vi "Measure Settings Dialog.vi"(8 "error in (no error)":errorcluster caption="错误输入（无错误）", 10 "测试类型":T1, 11 "Settings in":T5={"Hardware Configuration"={"电压读取设置"={"DAQmx Channel"="", "Max Input"=0.0, "Min Input"=0.0, "Sample Rate"=0.0, "Sample Number"=0, "DAQmx Task"="", "device in"=""}, "角度传感器设置"={"counter"="Dev1/ctr0", "units"=10146, "分辨率"=0, "初始角度"=0.0, "DecodingType"=10092, "A相端口"="/Dev1/PFI8", "B相端口"="/Dev1/PFI8", "task in"=""}}, "Logging Configuration"={"Log File Base Path"=path "", "电压传感器转换率"=[], "电压传感器本底"=[]}, "Action Configuration"={"PLC设置"={"ActLogicalStationNumber"=9600, "ActUtlType"=refnum}, "动作设置"={"自动跳法测试动作"={"夹紧"={"PLC指令"={"变量类型"=2, "PLC地址"=0, "size"=0, "写入数据(写入时有效)"=0}}, "通油"={"打开主阀"={"变量类型"=2, "PLC地址"=0, "size"=0, "写入数据(写入时有效)"=0}, "打开电磁阀"={"变量类型"=2, "PLC地址"=0, "size"=0, "写入数据(写入时有效)"=0}}, "压销"={"PLC指令"={"变量类型"=2, "PLC地址"=0, "size"=0, "写入数据(写入时有效)"=0}}}, "其他动作"={"其他指令1"={"变量类型"=2, "PLC地址"=0, "size"=0, "写入数据(写入时有效)"=0}, "其他指令2"={"变量类型"=2, "PLC地址"=0, "size"=0, "写入数据(写入时有效)"=0}, "其他指令3"={"变量类型"=2, "PLC地址"=0, "size"=0, "写入数据(写入时有效)"=0}, "其他指令4"={"变量类型"=2, "PLC地址"=0, "size"=0, "写入数据(写入时有效)"=0}, "其他指令5"={"变量类型"=2, "PLC地址"=0, "size"=0, "写入数据(写入时有效)"=0}}}, "电机设置"={"counter"="Dev1/ctr0", "方向端口"="", "当前方向"=FALSE, "频率"=0.0, "DAQmx Task"=""}, "所有测试电机转动逻辑"={"啮合测试电机转动逻辑"={"反转判断条件1"={"传感器序号"=0, "条件"=enum."小于", "值"=0.0, "条件判断时间间隔"=0, "反转等待时长"=0}, "停止判断条件1"={"角度传感器序号"=0, "正转/反转"=enum."正转", "反转次数"=0, "停止角度"=0.0, "停止角度误差范围"=0.0}}, "退回测试电机转动逻辑"={"反转判断条件1"={"传感器序号"=0, "条件"=enum."小于", "值"=0.0, "条件判断时间间隔"=0, "反转等待时长"=0}, "停止判断条件1"={"角度传感器序号"=0, "正转/反转"=enum."正转", "反转次数"=0, "停止角度"=0.0, "停止角度误差范围"=0.0}}, "功能测试电机转动逻辑"={"反转判断条件1"={"传感器序号"=0, "条件"=enum."小于", "值"=0.0, "条件判断时间间隔"=0, "反转等待时长"=0}, "停止判断条件1"={"角度传感器序号"=0, "正转/反转"=enum."正转", "反转次数"=0, "停止角度"=0.0, "停止角度误差范围"=0.0}}, "力特性测试电机转动逻辑"={"反转判断条件1"={"传感器序号"=0, "条件"=enum."小于", "值"=0.0, "条件判断时间间隔"=0, "反转等待时长"=0}, "停止判断条件1"={"角度传感器序号"=0, "正转/反转"=enum."正转", "反转次数"=0, "停止角度"=0.0, "停止角度误差范围"=0.0}}, "自动调阀测试分中电机转动逻辑"={"反转判断条件1"={"传感器序号"=0, "条件"=enum."小于", "值"=0.0, "条件判断时间间隔"=0, "反转等待时长"=0}, "停止判断条件1"={"角度传感器序号"=0, "正转/反转"=enum."正转", "反转次数"=0, "停止角度"=0.0, "停止角度误差范围"=0.0}}, "自动调阀测试对中电机转动逻辑"={"反转判断条件1"={"传感器序号"=0, "条件"=enum."小于", "值"=0.0, "条件判断时间间隔"=0, "反转等待时长"=0}, "停止判断条件1"={"角度传感器序号"=0, "正转/反转"=enum."正转", "反转次数"=0, "停止角度"=0.0, "停止角度误差范围"=0.0}}}}} caption="设置" {"Action Configuration"."动作设置"."其他动作"."其他指令5"."变量类型" items=["X", "Y", "M", "D"]; "Action Configuration"."动作设置"."其他动作"."其他指令4"."变量类型" items=["X", "Y", "M", "D"]; "Action Configuration"."动作设置"."其他动作"."其他指令3"."变量类型" items=["X", "Y", "M", "D"]; "Action Configuration"."动作设置"."其他动作"."其他指令2"."变量类型" items=["X", "Y", "M", "D"]; "Action Configuration"."动作设置"."其他动作"."其他指令1"."变量类型" items=["X", "Y", "M", "D"]; "Action Configuration"."动作设置"."自动跳法测试动作"."压销"."PLC指令"."变量类型" items=["X", "Y", "M", "D"]; "Action Configuration"."动作设置"."自动跳法测试动作"."通油"."打开电磁阀"."变量类型" items=["X", "Y", "M", "D"]; "Action Configuration"."动作设置"."自动跳法测试动作"."通油"."打开主阀"."变量类型" items=["X", "Y", "M", "D"]; "Action Configuration"."动作设置"."自动跳法测试动作"."夹紧"."PLC指令"."变量类型" items=["X", "Y", "M", "D"]; "Hardware Configuration"."角度传感器设置"."DecodingType" items=["X1"=10090, "X2"=10091, "X4"=10092, "Two Pulse Counting"=10313]; "Hardware Configuration"."角度传感器设置"."units" items=["Degrees"=10146, "Radians"=10273, "Ticks"=10304, "From Custom Scale"=10065]}) -> (0 "error out":errorcluster caption="错误输出", 1 "Cancelled?":bool=TRUE caption="取消？", 2 "UI Refresh Needed?":bool caption="需要刷新UI？", 3 "Settings out":T5={"Hardware Configuration"={"电压读取设置"={"DAQmx Channel"="", "Max Input"=0.0, "Min Input"=0.0, "Sample Rate"=0.0, "Sample Number"=0, "DAQmx Task"="", "device in"=""}, "角度传感器设置"={"counter"="Dev1/ctr0", "units"=10146, "分辨率"=0, "初始角度"=0.0, "DecodingType"=10092, "A相端口"="/Dev1/PFI8", "B相端口"="/Dev1/PFI8", "task in"=""}}, "Logging Configuration"={"Log File Base Path"=path "", "电压传感器转换率"=[], "电压传感器本底"=[]}, "Action Configuration"={"PLC设置"={"ActLogicalStationNumber"=9600, "ActUtlType"=refnum}, "动作设置"={"自动跳法测试动作"={"夹紧"={"PLC指令"={"变量类型"=2, "PLC地址"=0, "size"=0, "写入数据(写入时有效)"=0}}, "通油"={"打开主阀"={"变量类型"=2, "PLC地址"=0, "size"=0, "写入数据(写入时有效)"=0}, "打开电磁阀"={"变量类型"=2, "PLC地址"=0, "size"=0, "写入数据(写入时有效)"=0}}, "压销"={"PLC指令"={"变量类型"=2, "PLC地址"=0, "size"=0, "写入数据(写入时有效)"=0}}}, "其他动作"={"其他指令1"={"变量类型"=2, "PLC地址"=0, "size"=0, "写入数据(写入时有效)"=0}, "其他指令2"={"变量类型"=2, "PLC地址"=0, "size"=0, "写入数据(写入时有效)"=0}, "其他指令3"={"变量类型"=2, "PLC地址"=0, "size"=0, "写入数据(写入时有效)"=0}, "其他指令4"={"变量类型"=2, "PLC地址"=0, "size"=0, "写入数据(写入时有效)"=0}, "其他指令5"={"变量类型"=2, "PLC地址"=0, "size"=0, "写入数据(写入时有效)"=0}}}, "电机设置"={"counter"="Dev1/ctr0", "方向端口"="", "当前方向"=FALSE, "频率"=0.0, "DAQmx Task"=""}, "所有测试电机转动逻辑"={"啮合测试电机转动逻辑"={"反转判断条件1"={"传感器序号"=0, "条件"=enum."小于", "值"=0.0, "条件判断时间间隔"=0, "反转等待时长"=0}, "停止判断条件1"={"角度传感器序号"=0, "正转/反转"=enum."正转", "反转次数"=0, "停止角度"=0.0, "停止角度误差范围"=0.0}}, "退回测试电机转动逻辑"={"反转判断条件1"={"传感器序号"=0, "条件"=enum."小于", "值"=0.0, "条件判断时间间隔"=0, "反转等待时长"=0}, "停止判断条件1"={"角度传感器序号"=0, "正转/反转"=enum."正转", "反转次数"=0, "停止角度"=0.0, "停止角度误差范围"=0.0}}, "功能测试电机转动逻辑"={"反转判断条件1"={"传感器序号"=0, "条件"=enum."小于", "值"=0.0, "条件判断时间间隔"=0, "反转等待时长"=0}, "停止判断条件1"={"角度传感器序号"=0, "正转/反转"=enum."正转", "反转次数"=0, "停止角度"=0.0, "停止角度误差范围"=0.0}}, "力特性测试电机转动逻辑"={"反转判断条件1"={"传感器序号"=0, "条件"=enum."小于", "值"=0.0, "条件判断时间间隔"=0, "反转等待时长"=0}, "停止判断条件1"={"角度传感器序号"=0, "正转/反转"=enum."正转", "反转次数"=0, "停止角度"=0.0, "停止角度误差范围"=0.0}}, "自动调阀测试分中电机转动逻辑"={"反转判断条件1"={"传感器序号"=0, "条件"=enum."小于", "值"=0.0, "条件判断时间间隔"=0, "反转等待时长"=0}, "停止判断条件1"={"角度传感器序号"=0, "正转/反转"=enum."正转", "反转次数"=0, "停止角度"=0.0, "停止角度误差范围"=0.0}}, "自动调阀测试对中电机转动逻辑"={"反转判断条件1"={"传感器序号"=0, "条件"=enum."小于", "值"=0.0, "条件判断时间间隔"=0, "反转等待时长"=0}, "停止判断条件1"={"角度传感器序号"=0, "正转/反转"=enum."正转", "反转次数"=0, "停止角度"=0.0, "停止角度误差范围"=0.0}}}}} caption="设置" {"Action Configuration"."动作设置"."其他动作"."其他指令5"."变量类型" items=["X", "Y", "M", "D"]; "Action Configuration"."动作设置"."其他动作"."其他指令4"."变量类型" items=["X", "Y", "M", "D"]; "Action Configuration"."动作设置"."其他动作"."其他指令3"."变量类型" items=["X", "Y", "M", "D"]; "Action Configuration"."动作设置"."其他动作"."其他指令2"."变量类型" items=["X", "Y", "M", "D"]; "Action Configuration"."动作设置"."其他动作"."其他指令1"."变量类型" items=["X", "Y", "M", "D"]; "Action Configuration"."动作设置"."自动跳法测试动作"."压销"."PLC指令"."变量类型" items=["X", "Y", "M", "D"]; "Action Configuration"."动作设置"."自动跳法测试动作"."通油"."打开电磁阀"."变量类型" items=["X", "Y", "M", "D"]; "Action Configuration"."动作设置"."自动跳法测试动作"."通油"."打开主阀"."变量类型" items=["X", "Y", "M", "D"]; "Action Configuration"."动作设置"."自动跳法测试动作"."夹紧"."PLC指令"."变量类型" items=["X", "Y", "M", "D"]; "Hardware Configuration"."角度传感器设置"."DecodingType" items=["X1"=10090, "X2"=10091, "X4"=10092, "Two Pulse Counting"=10313]; "Hardware Configuration"."角度传感器设置"."units" items=["Degrees"=10146, "Radians"=10273, "Ticks"=10304, "From Custom Scale"=10065]})   [LabVIEW 2015, in "Settings.lvlib"]
doc: "用于选择用户设置的对话框。"
uses:
  Settings.lvlib
  <vilib>/Utility/xml.llb/Write to XML File(string).vi
  Acquisition/Hardware Configuration.ctl
  Acquisition/Acquisition.lvlib
  Logging/Logging Configuration.ctl
  Logging/Logging.lvlib
  Settings.ctl
  Action/Action.lvlib
  Measure/Measure Type.ctl
  Action/Hardware Configuration.ctl
panel:
  in  "电机转动逻辑1":T2
  in  "Cancel Button":bool caption="取消按钮"
  in  "OK Button":bool caption="确定按钮"
  # "电机转动设置"
  # "对话框不可见部分（用于连线板）"
  # "1、扭矩\n\n2、油压\n\n3、左推力\n\n4、右推力\n\n5、流量\n\n6、位移量"
  # "1、扭矩\n\n2、油压\n\n3、左推力\n\n4、右推力\n\n5、流量\n\n6、位移量"
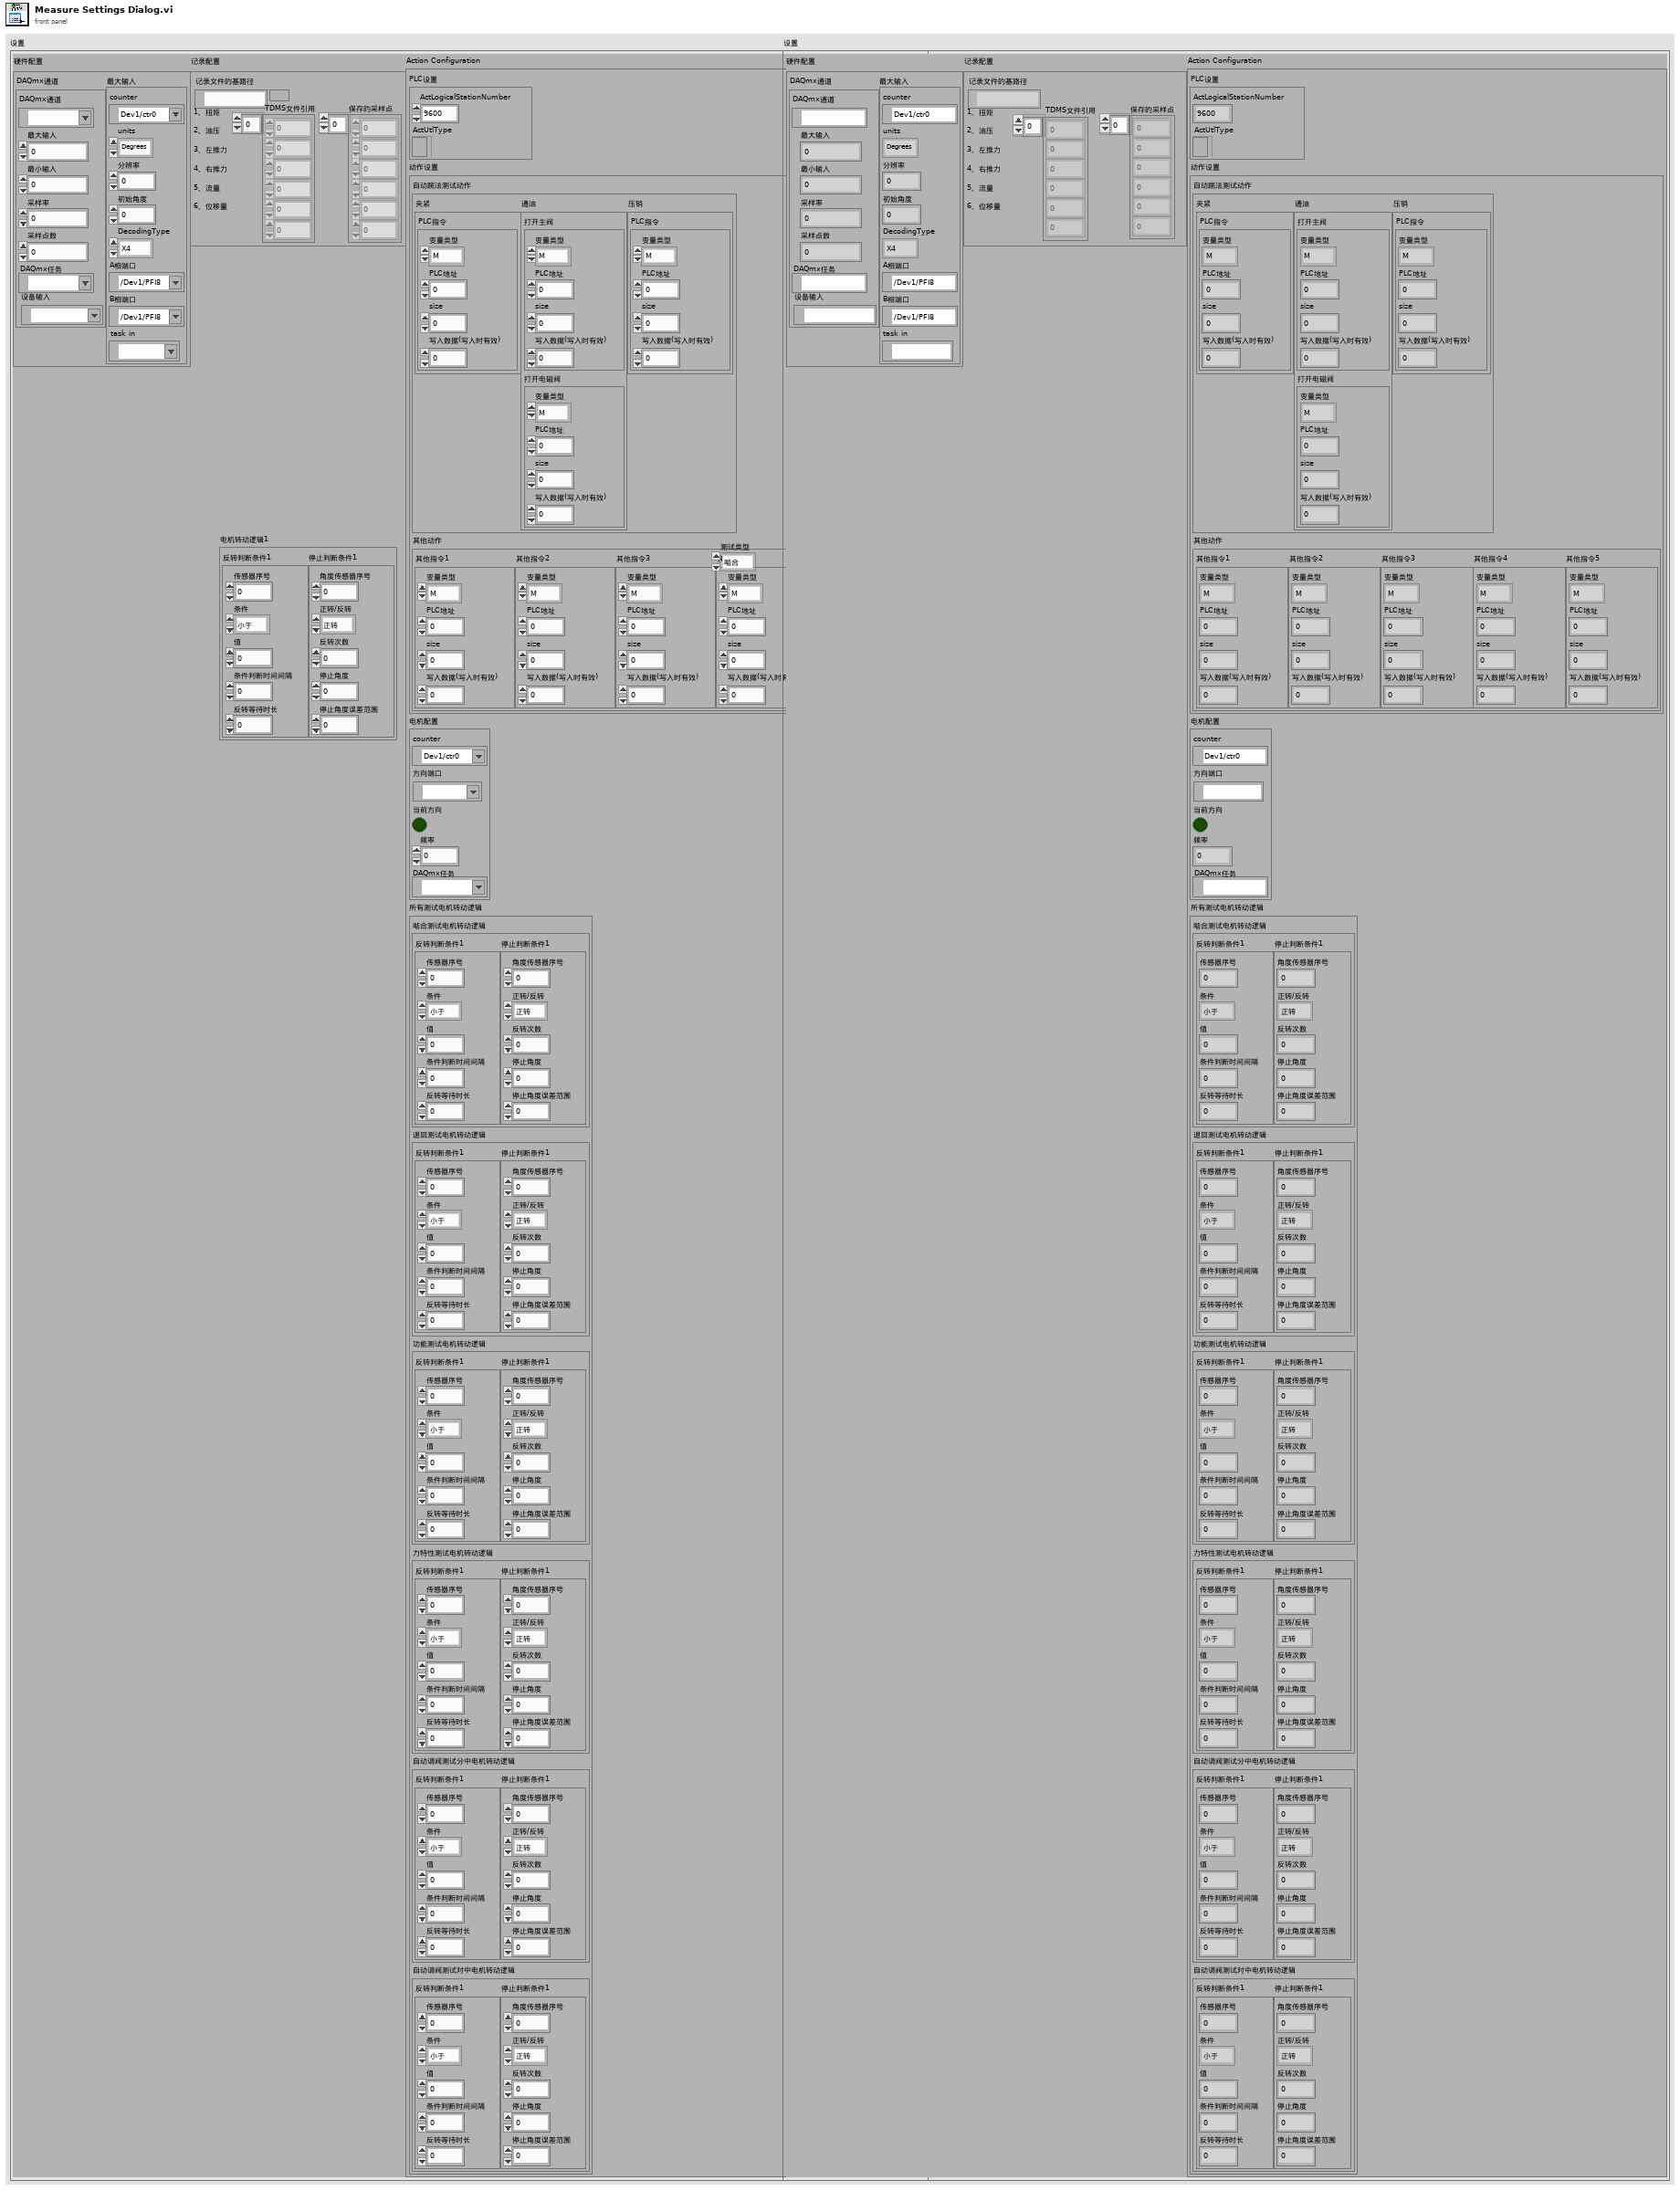
[diagram p1: front panel]
types:
  T1 = typedef "Measure Type.ctl" = enum16{"啮合", "退回", "功能", "力特性", "内泄漏", "自动调阀测试"}
  T2 = typedef "Action.lvlib/电机转动逻辑1.ctl" = cluster{"反转判断条件1":T3, "停止判断条件1":T4}
  T3 = typedef "Action.lvlib/反转判断条件1.ctl" = cluster{"传感器序号":i32, "条件":enum16{"小于", "大于", "等于"}, "值":dbl, "条件判断时间间隔":i32, "反转等待时长":i32}
  T4 = typedef "Action.lvlib/停止判断条件1.ctl" = cluster{"角度传感器序号":i32, "正转/反转":enum16{"正转", "反转"}, "反转次数":i32, "停止角度":dbl, "停止角度误差范围":dbl}
  T5 = typedef "Settings.lvlib/Settings.ctl" = cluster{"Hardware Configuration":T6, "Logging Configuration":T7, "Action Configuration":T8}
  T6 = typedef "Acquisition.lvlib/Hardware Configuration.ctl" = cluster{"电压读取设置":cluster{"DAQmx Channel":tag, "Max Input":dbl, "Min Input":dbl, "Sample Rate":dbl, "Sample Number":i32, "DAQmx Task":refnum<k21>, "device in":tag}, "角度传感器设置":cluster{"counter":tag, "units":i32, "分辨率":i32, "初始角度":dbl, "DecodingType":i32, "A相端口":tag, "B相端口":tag, "task in":refnum<k21>}}
  T7 = typedef "Logging.lvlib/Logging Configuration.ctl" = cluster{"Log File Base Path":path, "电压传感器转换率":dbl[], "电压传感器本底":dbl[]}
  T8 = typedef "Action.lvlib/Hardware Configuration.ctl" = cluster{"PLC设置":T9, "动作设置":T10, "电机设置":T14, "所有测试电机转动逻辑":T15}
  T9 = typedef "Action.lvlib/PLC设置.ctl" = cluster{"ActLogicalStationNumber":i32, "ActUtlType":refnum<k7>}
  T10 = typedef "Action.lvlib/动作设置.ctl" = cluster{"自动跳法测试动作":T11, "其他动作":T13}
  T11 = typedef "Action.lvlib/自动调阀测试动作设置.ctl" = cluster{"夹紧":cluster{"PLC指令":T12}, "通油":cluster{"打开主阀":T12, "打开电磁阀":T12}, "压销":cluster{"PLC指令":T12}}
  T12 = typedef "Action.lvlib/PLC控制指令.ctl" = cluster{"变量类型":u32, "PLC地址":i32, "size":i32, "写入数据(写入时有效)":i16}
  T13 = typedef "Action.lvlib/其他动作设置 .ctl" = cluster{"其他指令1":T12, "其他指令2":T12, "其他指令3":T12, "其他指令4":T12, "其他指令5":T12}
  T14 = typedef "Action.lvlib/电机控制设置.ctl" = cluster{"counter":tag, "方向端口":tag, "当前方向":bool, "频率":dbl, "DAQmx Task":refnum<k21>}
  T15 = typedef "Action.lvlib/所有测试电机转动逻辑.ctl" = cluster{"啮合测试电机转动逻辑":T2, "退回测试电机转动逻辑":T2, "功能测试电机转动逻辑":T2, "力特性测试电机转动逻辑":T2, "自动调阀测试分中电机转动逻辑":T2, "自动调阀测试对中电机转动逻辑":T2}
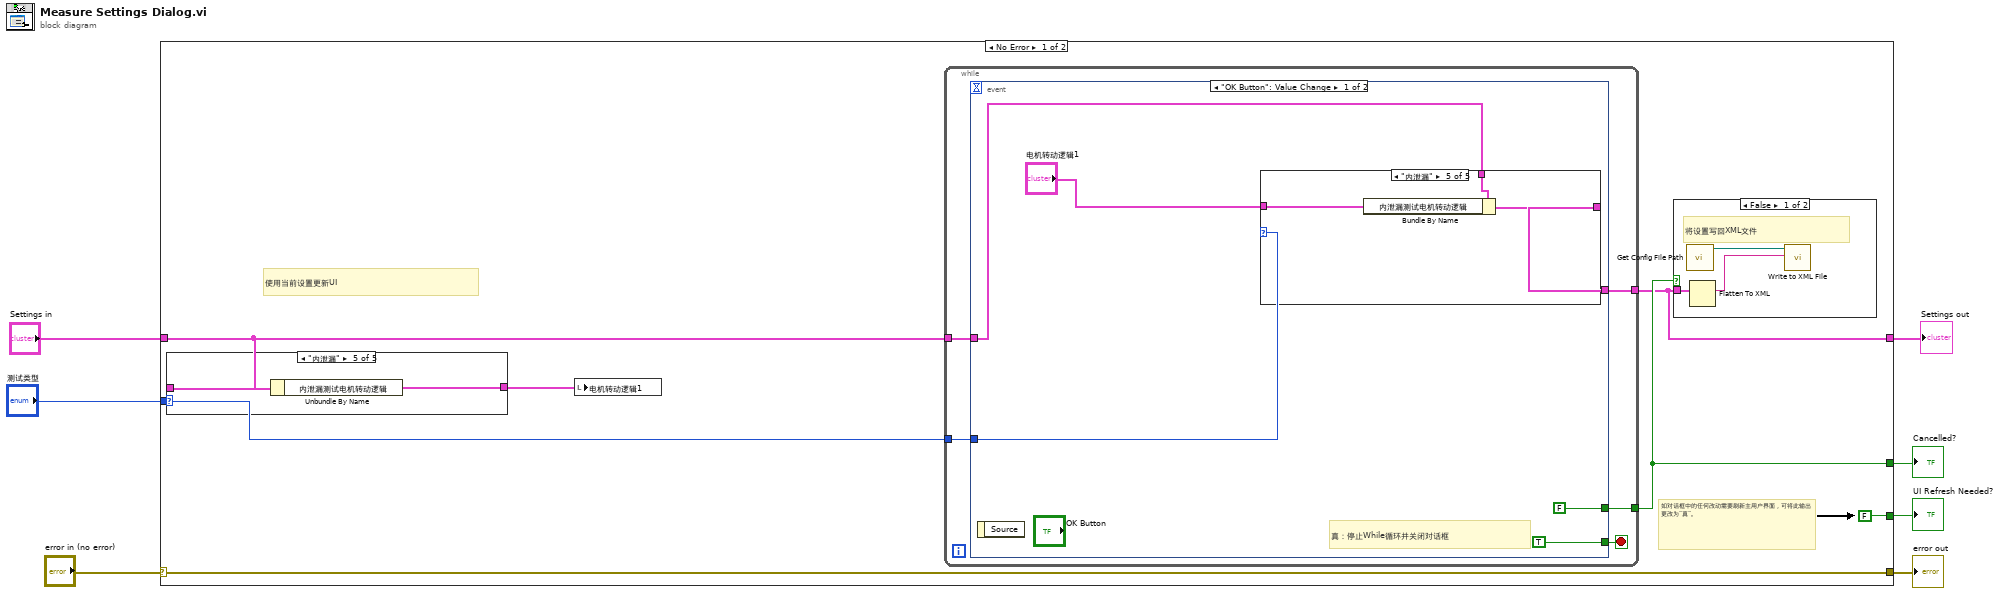
[diagram p0: block diagram]
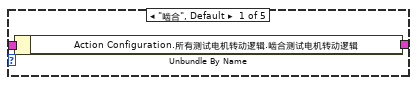
[diagram p2: hidden frame]
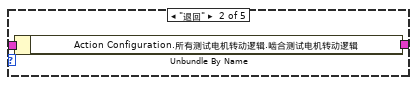
[diagram p3: hidden frame]
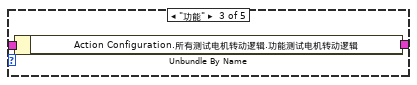
[diagram p4: hidden frame]
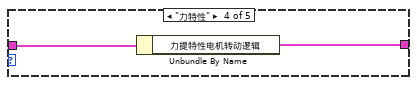
[diagram p5: hidden frame]
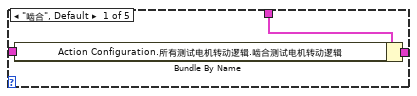
[diagram p6: hidden frame]
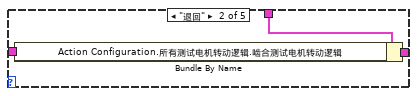
[diagram p7: hidden frame]
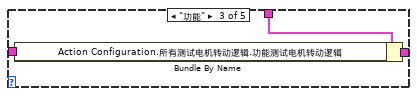
[diagram p8: hidden frame]
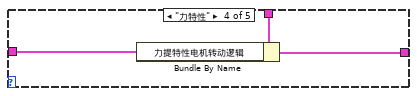
[diagram p9: hidden frame]
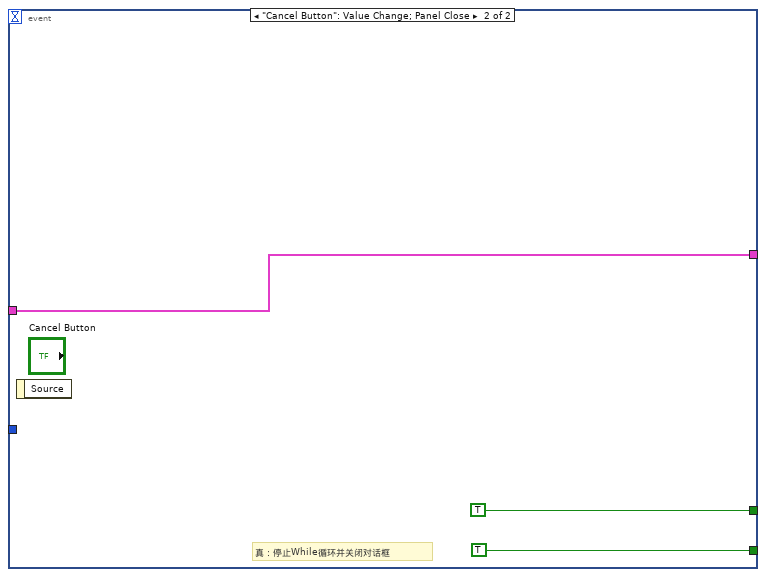
[diagram p10: hidden frame]
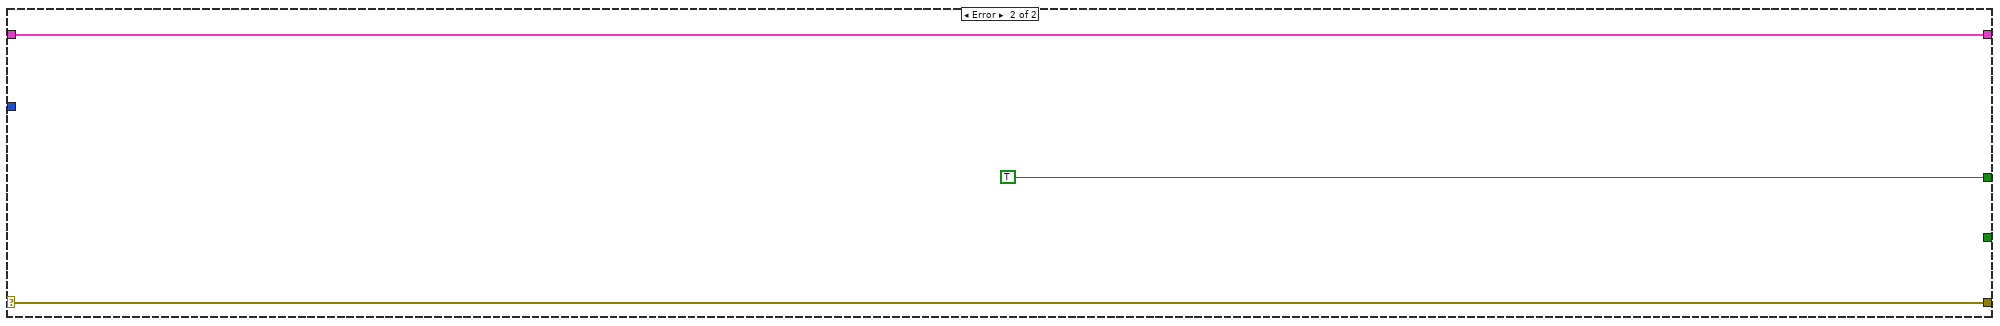
[diagram p12: hidden frame]
diagram:
  n1 = case shown="No Error" "error in (no error)" {
    selector: "error in (no error)" -> [w14 w59]
    tunnel: [w14 w59] -> w7
    tunnel: "Settings in" -> [w10 w58]
    tunnel: [w11 w58] -> w2
    tunnel: [FALSE ("UI Refresh Needed?") _] -> w6
    tunnel: [w12 TRUE ("UI Refresh Needed?")] -> w5
    tunnel: "测试类型" -> [w8 _]
    frame No Error {
      # "使用当前设置更新UI"
      # "如对话框中的任何改动需要刷新主用户界面，可将此输出更改为“真”。"
      n2 = case shown="\"内泄漏\"" w8 {
        tunnel: w10 -> [w16 w18 w20 w22 w24]
        tunnel: [w15 w17 w19 w21 w23] -> w9
        frame "啮合", Default {
          n3 = Unbundle By Name(w16) -> ("Action Configuration.所有测试电机转动逻辑.啮合测试电机转动逻辑"=w15:T2)
        }
        frame "退回" {
          n4 = Unbundle By Name(w18) -> ("Action Configuration.所有测试电机转动逻辑.啮合测试电机转动逻辑"=w17:T2)
        }
        frame "功能" {
          n5 = Unbundle By Name(w20) -> ("Action Configuration.所有测试电机转动逻辑.功能测试电机转动逻辑"=w19:T2)
        }
        frame "力特性" {
          n6 = Unbundle By Name(w22) -> ("力提特性电机转动逻辑"=w21:T2)
        }
        frame "内泄漏" {
          n7 = Unbundle By Name(w24) -> ("内泄漏测试电机转动逻辑"=w23:T2)
        }
      }
      n8 = local write "电机转动逻辑1"(w9) -> ()
      n9 = while {
        tunnel: [w29] -> w12
        tunnel: [w28] -> w11
        tunnel: w10 -> [w27]
        tunnel: w8 -> [w25]
        stop <- w26 stop-if-true
        n10 = event shown="[0] \"OK Button\": Value Change" {
          selector: _ -> [_ _]
          dyn-events: _ -> [_ _]
          timeout: _ -> [_ _]
          tunnel: [w33 w53] -> w28
          tunnel: w27 -> [w32 w53]
          tunnel: [FALSE ("UI Refresh Needed?") TRUE ("UI Refresh Needed?")] -> w29
          tunnel: [TRUE TRUE] -> w26
          tunnel: w25 -> [w30 _]
          event "OK Button": Value Change {
            # "真：停止While循环并关闭对话框"
            n11 = event-data() -> ()  [unwired: 1 in, 1 out]
            n12 = case shown="\"内泄漏\"" w30 {
              tunnel: [w38 w41 w44 w47 w50] -> w33
              tunnel: w32 -> [w37 w40 w43 w46 w49]
              tunnel: "电机转动逻辑1" -> [w36 w39 w42 w45 w48]
              frame "啮合", Default {
                n13 = Bundle By Name(cluster=w37, "Action Configuration.所有测试电机转动逻辑.啮合测试电机转动逻辑"=w36) -> (w38:T5)
              }
              frame "退回" {
                n14 = Bundle By Name(cluster=w40, "Action Configuration.所有测试电机转动逻辑.啮合测试电机转动逻辑"=w39) -> (w41:T5)
              }
              frame "功能" {
                n15 = Bundle By Name(cluster=w43, "Action Configuration.所有测试电机转动逻辑.功能测试电机转动逻辑"=w42) -> (w44:T5)
              }
              frame "力特性" {
                n16 = Bundle By Name(cluster=w46, "力提特性电机转动逻辑"=w45) -> (w47:T5)
              }
              frame "内泄漏" {
                n17 = Bundle By Name(cluster=w49, "内泄漏测试电机转动逻辑"=w48) -> (w50:T5)
              }
            }
          }
          event "Cancel Button": Value Change; Panel Close {
            # "真：停止While循环并关闭对话框"
            n18 = event-data() -> ()  [unwired: 1 in, 1 out]
          }
        }
      }
      n19 = case shown="False" w12 {
        tunnel: w11 -> [w55 _]
        frame False {
          # "将设置写回XML文件"
          n20 = call "Get Config File Path.vi"() -> ("XML File Path"=w56:path)  [unwired: 10 in, 1 out]
          n21 = Flatten To XML(anything=w55) -> (xml string=w54:string)
          n22 = call-poly <vilib>:"Write to XML File.vi"("XML Input"=w54, "XML File Path"=w56) -> ()  [unwired: 7 in, 3 out]
        }
        frame True {
        }
      }
    }
    frame Error {
    }
  }
  "UI Refresh Needed?" <- w6
  "error out" <- w7
  "Cancelled?" <- w5
  "Settings out" <- w2
